vi "grow tx data.vi"(1 "value":dbl, 2 "time":dbl, 3 "tx data in":cluster{"t":dbl[], "x":dbl[]}) -> (0 "tx data out":cluster{"t":dbl[], "x":dbl[]})   [LabVIEW 2010]
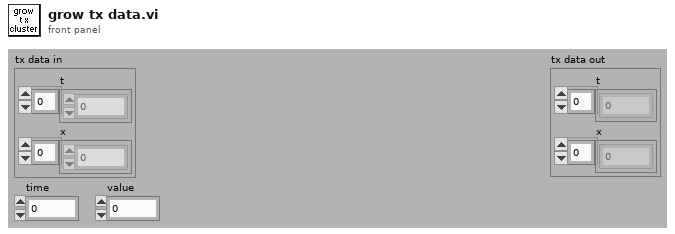
[diagram p1: front panel]
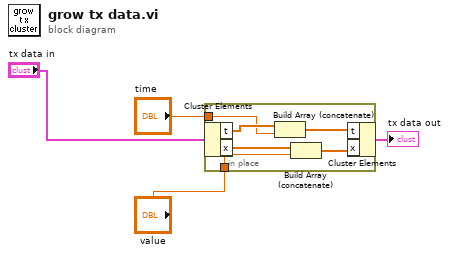
[diagram p0: block diagram]
diagram:
  n1 = in-place {
    in-place-border: "time" -> [w9]
    in-place-border: "value" -> [w7]
    n2 = in-place-cluster #1("tx data in") -> ("t"=w10:dbl[], "x"=w8:dbl[])
    n3 = Build Array (concatenate)(w10, w9) -> (w6:dbl[])
    n4 = Build Array (concatenate)(w8, w7) -> (w5:dbl[])
    n5 = in-place-cluster #1("t"=w6, "x"=w5) -> (→"tx data out":cluster{"t":dbl[], "x":dbl[]})
  }
